vi "Write Enable Output Status (Single).vi"(8 "error in":errorcluster, 9 "Channel Index":i32=1, 10 "Enable Output":bool, 11 "Cycler in":refnum<class "Cycler.lvclass">) -> (0 "error out":errorcluster, 3 "Cycler out":refnum<class "Cycler.lvclass">)   [LabVIEW 2023, in "Cycler.lvclass"]
uses:
  Cycler.lvclass
  Cycler.lvclass/Cycler.ctl
  <vilib>/ADAS Replay HIL/Channels/Tag Wrapper/Tag Wrapper.lvlib
  <vilib>/ADAS Replay HIL/Channels/Tag Wrapper/Polymorphic/Write Channel (Boolean).vi
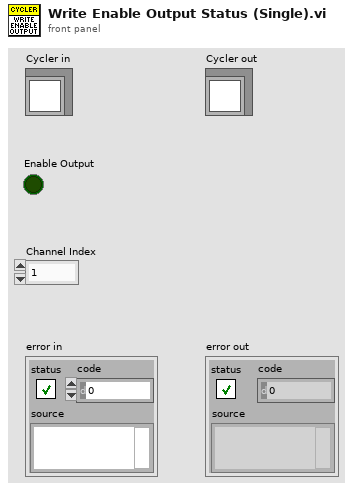
[diagram p1: front panel]
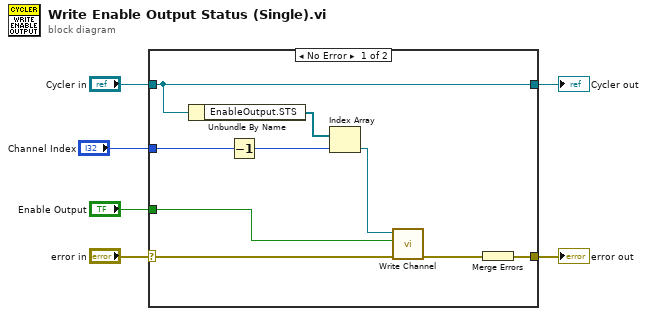
[diagram p0: block diagram]
diagram:
  n1 = case shown="No Error" "error in" {
    selector: "error in" -> [w15 w16]
    tunnel: [w10 w16] -> w5
    tunnel: [w13 w17] -> w3
    tunnel: "Cycler in" -> [w13 w17]
    tunnel: "Enable Output" -> [w11 _]
    tunnel: "Channel Index" -> [w8 _]
    frame No Error {
      n2 = Unbundle By Name(w13) -> ("EnableOutput.STS"=w12:refnum<k21>[])
      n3 = Decrement(x=w8) -> (x-1=w7:i32)
      n4 = Index Array(array=w12, index=w7) -> (element=w9:refnum<k21>)
      n5 = call-poly <vilib>:"Write Channel.vi"("error in"=w15, "Value to Write"=w11, "ADAS HIL Channel in"=w9) -> ("error out"=w14:errorcluster)  [unwired: 6 in, 2 out]
      n6 = Merge Errors(w14) -> (w10:errorcluster)
    }
    frame Error {
    }
  }
  "error out" <- w5
  "Cycler out" <- w3
